vi "sineWave.vi"(4 "phase":dbl, 6 "samples":i32, 7 "duration":dbl, 8 "error in (no error)":errorcluster, 9 "amplitude":dbl, 10 "freq":dbl, 11 "SoundDeviceData in":refnum<class "SoundDeviceData.lvclass">) -> (0 "error out":errorcluster, 1 "phase out":dbl, 2 "sine wave":dbl[](array[numeric]), 3 "SoundDeviceData out":refnum<class "SoundDeviceData.lvclass">)   [LabVIEW 2009, in "DataMappers.lvlib" / "SoundDeviceData.lvclass"]
uses:
  SoundDeviceData.lvclass
  <vilib>/Analysis/NI_AALBase.lvlib
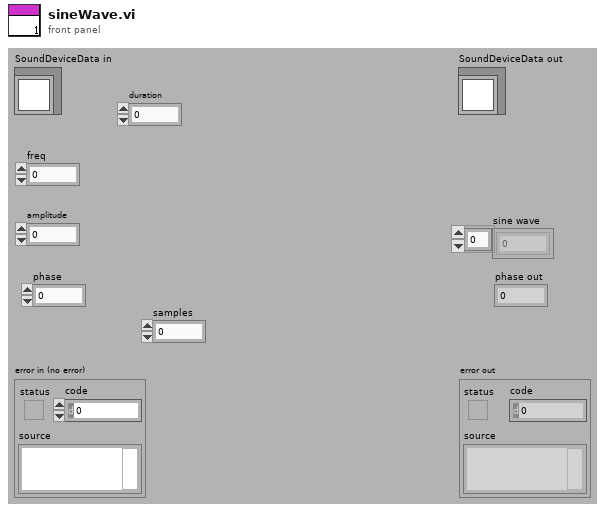
[diagram p1: front panel]
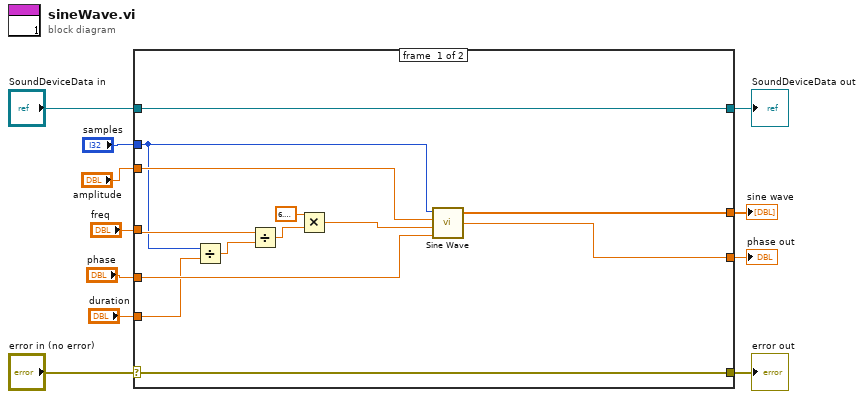
[diagram p0: block diagram]
diagram:
  n1 = case shown="No Error" "error in (no error)" {
    selector: "error in (no error)" -> [w23 w26]
    tunnel: [w23 w26] -> w10
    tunnel: [w24 w25] -> w8
    tunnel: "SoundDeviceData in" -> [w24 w25]
    tunnel: "samples" -> [w15 _]
    tunnel: "amplitude" -> [w22 _]
    tunnel: "freq" -> [w19 _]
    tunnel: "phase" -> [w21 _]
    tunnel: [w20 _] -> w1
    tunnel: "duration" -> [w17 _]
    tunnel: [w14 _] -> w2
    frame #0 {
      n2 = Divide(x=w15, y=w17) -> (x/y=w16:dbl)
      n3 = Divide(x=w19, y=w16) -> (x/y=w18:dbl)
      n4 = Multiply(x=6.283185307179586, y=w18) -> (x*y=w13:dbl)
      n5 = call <vilib>:"Sine Wave.vi"("samples"=w15, "amplitude"=w22, "frequency"=w13, "phase in"=w21) -> ("sine wave"=w20:dbl[], "phase out"=w14:dbl)  [unwired: 1 in, 1 out]
    }
    frame #1 {
    }
  }
  "error out" <- w10
  "SoundDeviceData out" <- w8
  "phase out" <- w2
  "sine wave" <- w1
